vi "Import Channels.vi"(8 "error in":errorcluster, 11 "Objects in":T1) -> (0 "error out":errorcluster, 3 "Objects out":T1)   [LabVIEW 2014, in "FPGA Module editor node.lvclass"]
uses:
  FPGA Module editor node.lvclass
  module/configuration/FPGA Module configuration.lvclass
  fpga channel/FPGA Channel.lvclass
  module/configuration/Line.ctl
  <vilib>/NI/DCAF/Tag Editor Core/Configuration Editor/Classes/Module editor node/module editor node.lvclass
  <vilib>/NI/Module Execution Interface/Engine Configuration/engine configuration.lvclass
  <vilib>/NI/Configuration Framework/serializable configuration/NISE_CEF_serializable configuration.lvclass
  <vilib>/NI/DCAF/Tag Editor Core/Configuration Editor/Classes/Engine Parent/Engine Parent Editor Node.lvclass
  <vilib>/NI/DCAF/Tag Editor Core/Table API/Table Manager/object ref.ctl
  <vilib>/NI/DCAF/Tag Editor Core/Table API/Table Manager/Table Manager.lvclass
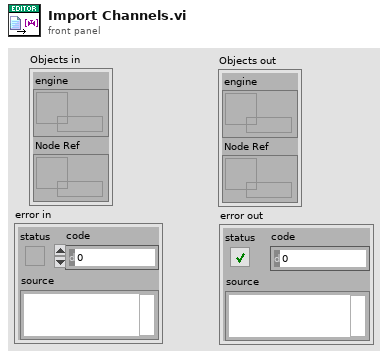
[diagram p1: front panel]
types:
  T1 = typedef "Table Manager.lvlib/Table Manager.lvclass/object ref.ctl" = cluster{"engine":refnum<data-value>, "Node Ref":refnum<data-value>}
  T2 = typedef "FPGA Module configuration.lvclass/Line.ctl" = cluster{"Channel":refnum<class "FPGA Channel.lvclass">}
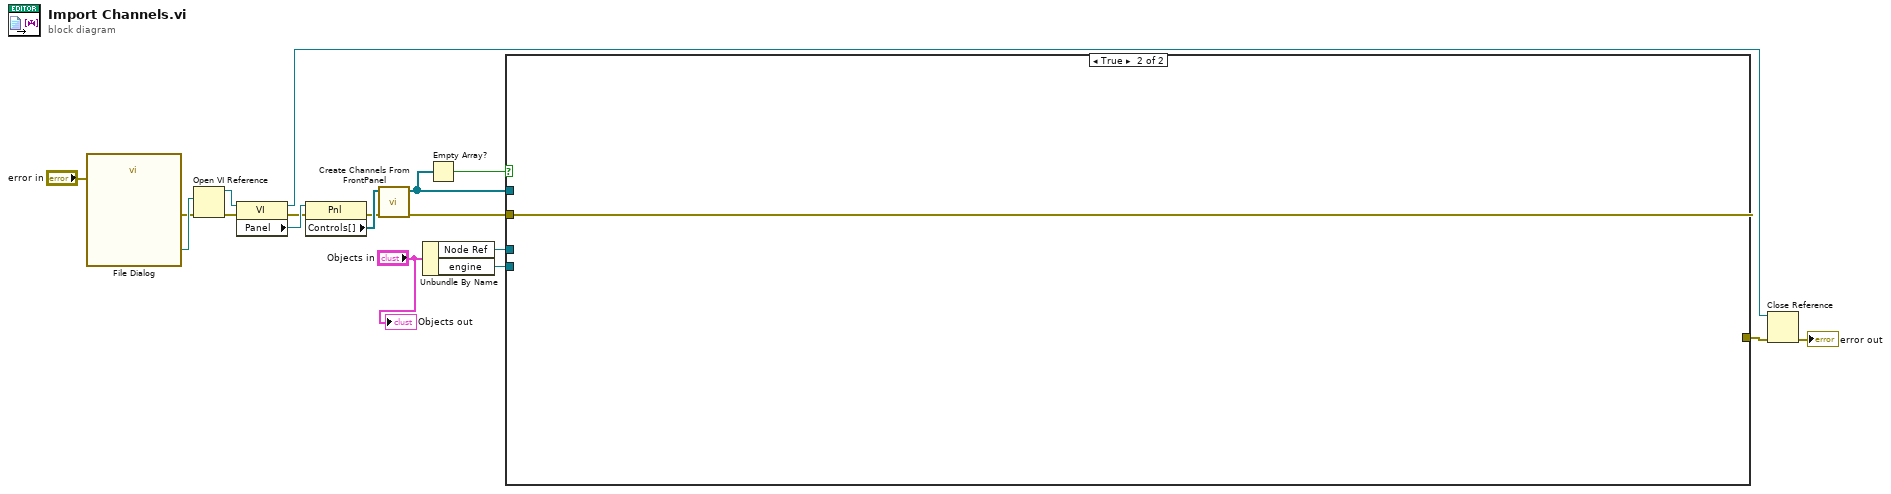
[diagram p0: block diagram]
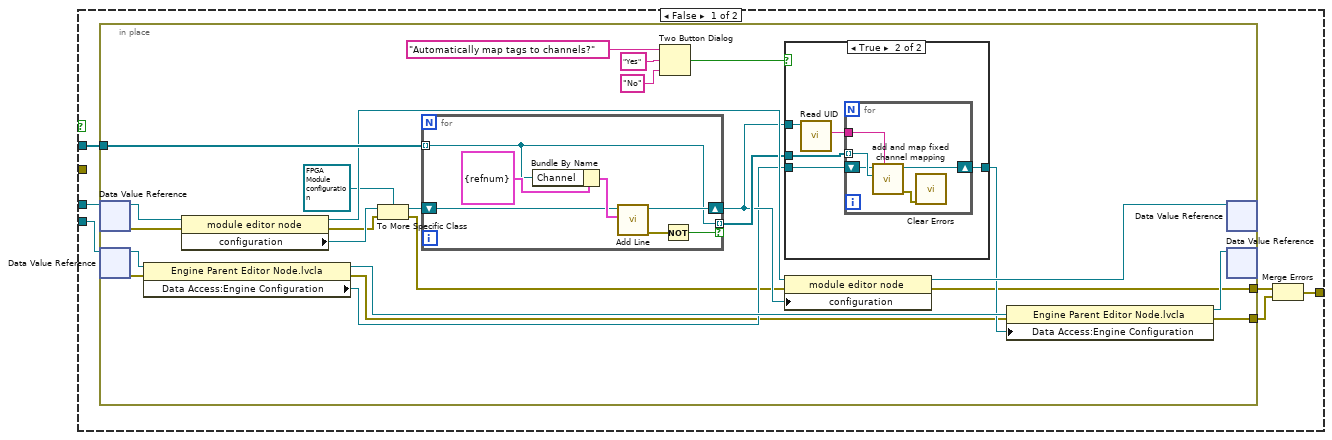
[diagram p2: hidden frame]
diagram:
  n1 = call "File Dialog"("error in"="error in") -> ("selected path"=w18:path, "error out"=w12:errorcluster)  [unwired: 11 in, 2 out]
  n2 = Open VI Reference(vi path=w18, error in (no error)=w12) -> (vi reference=w17:refnum<vi>, error out=w14:errorcluster)  [unwired: 4 in]
  n3 = property class="VI"(reference=w17, error in=w14) -> (reference out=w5:refnum<vi>, error out=w13:errorcluster, "Panel"=w16:refnum<vi>)
  n4 = property class="Pnl"(reference=w16, error in=w13) -> (error out=w11:errorcluster, "Controls[]"=w15:refnum<vi>[])  [unwired: 1 out]
  n5 = call "Create Channels From FrontPanel.vi"("error in (no error)"=w11, "Controls[]"=w15) -> ("error out"=w9:errorcluster, "Array"=w8:refnum<class "FPGA Channel.lvclass">[])  [unwired: 8 in]
  n6 = Unbundle By Name("Objects in") -> ("Node Ref"=w7:refnum<data-value>, "engine"=w6:refnum<data-value>)
  n7 = Empty Array?(array=w8) -> (empty?=w10:bool)
  n8 = case shown="True" w10 {
    tunnel: w9 -> [_ w68]
    tunnel: w8 -> [w24 _]
    tunnel: w7 -> [w23 _]
    tunnel: w6 -> [w22 _]
    tunnel: [w19 w68] -> w4
    frame False {
      n9 = in-place {
        in-place-border: w24 -> [w49]
        in-place-border: [w26] -> w21
        in-place-border: [w25] -> w20
        n10 = in-place-dvr #1(w23) -> (w48:refnum<class "module editor node.lvclass">, w32:errorcluster)
        n11 = in-place-dvr #2(w22) -> (w47:refnum<class "Engine Parent Editor Node.lvclass">, w31:errorcluster)
        n12 = property class="Engine Parent Editor Node.lvcla"(reference=w47, error in=w31) -> (reference out=w44:refnum<class "Engine Parent Editor Node.lvclass">, error out=w27:errorcluster, "Data Access:Engine Configuration"=w30:refnum<class "engine configuration.lvclass">)
        n13 = property class="module editor node"(reference=w48, error in=w32) -> (reference out=w45:refnum<class "module editor node.lvclass">, error out=w39:errorcluster, "configuration"=w46:refnum<class "NISE_CEF_serializable configuration.lvclass">)
        n14 = To More Specific Class(target class=refnum<class "FPGA Module configuration.lvclass"> refnum ("FPGA Module configuration"), reference=w46, error in=w39) -> (specific class reference=w41:refnum<class "FPGA Module configuration.lvclass">, error out=w28:errorcluster)
        n15 = for {
          tunnel: w49 -> [w62] mode=indexing
          shift-right: [w64] -> w33
          shift-left: w41 -> [w65]
          tunnel: [w62] -> w34 mode=indexing if=w61
          n16 = Bundle By Name(cluster=T2 {"Channel"=refnum} ("Line"), "Channel"=w62) -> (w66:T2)
          n17 = call "Add Line.vi"("Line"=w66, "FPGA Module configuration in"=w65) -> ("error out"=w63:errorcluster, "FPGA Module configuration out"=w64:refnum<class "FPGA Module configuration.lvclass">)  [unwired: 7 in, 1 out]
          n18 = Not(x=w63) -> (.not. x?=w61:bool)
        }
        n19 = Two Button Dialog(message="Automatically map tags to channels?", 1:"No" ("F button name (\"Cancel\")"), 2:"Yes" ("T button name (\"OK\")")) -> (T button?=w35:bool)
        n20 = case shown="True" w35 {
          tunnel: w34 -> [_ w55]
          tunnel: w33 -> [_ w54]
          tunnel: w30 -> [w50 w52]
          tunnel: [w50 w51] -> w29
          frame False {
          }
          frame True {
            n21 = call <vilib>:"Read UID.vi"("configuration in"=w54) -> ("instance id"=w53:string)  [unwired: 8 in, 2 out]
            n22 = for {
              tunnel: w55 -> [w59] mode=indexing
              tunnel: w53 -> [w60]
              shift-right: [w57] -> w51
              shift-left: w52 -> [w56]
              n23 = call <vilib>:"add and map fixed channel mapping.vi"("module instance"=w60, "fixed channel"=w59, "engine configuration in"=w56) -> ("error out"=w58:errorcluster, "engine configuration out"=w57:refnum<class "engine configuration.lvclass">)  [unwired: 7 in]
              n24 = call <vilib>:"Clear Errors.vi"("error in (no error)"=w58) -> ()  [unwired: 5 in, 2 out]
            }
          }
        }
        n25 = property class="module editor node"(reference=w45, error in=w28, "configuration"=w33) -> (reference out=w42:refnum<class "module editor node.lvclass">, error out=w26:errorcluster)
        n26 = property class="Engine Parent Editor Node.lvcla"(reference=w44, error in=w27, "Data Access:Engine Configuration"=w29) -> (reference out=w43:refnum<class "Engine Parent Editor Node.lvclass">, error out=w25:errorcluster)
        n27 = in-place-dvr #1(w42) -> ()  [unwired: 2 out]
        n28 = in-place-dvr #2(w43) -> ()  [unwired: 2 out]
      }
      n29 = Merge Errors(w21, w20) -> (w19:errorcluster)
    }
    frame True {
    }
  }
  n30 = Close Reference(reference=w5, error in (no error)=w4) -> (error out=→"error out":errorcluster)
  "Objects out" <- "Objects in"
